vi "FPGA Main Default.vi"() -> (0 "ENC.B.CNTR 2":u32)   [LabVIEW 2017]
doc: "The myRIO v1.1 FPGA Shipping Personality. This personality contains support for:\n- 2 Analog Input Interrupt channel\n- 4 Digital Input Interrupt channel\n- 1 Timer\n- 1 Accelerometer\n- 1 Button\n- 4 LED\n- 10 Analog Input channels with 1 Sample\n- 6 Analog Output channels with 1 Sample\n- 40 Digital I/O channels with 1 Sample\n- 2 I2C channels\n- 4 Encoder channels\n- 6 PWM channels\n- 2 SPI channels"
uses:
  Sub VIs/Utilities/Start Boolean.ctl
  <vilib>/Platform/TimedLoop/XDataNode/timing_clust.ctl
  <vilib>/Platform/TimedLoop/XDataNode/nitl_modes.ctl
  <vilib>/Platform/TimedLoop/XDataNode/wakeup.ctl
  <vilib>/rvi/Emulation/niFpgaGetClockAttributes.vi
  <vilib>/rvi/Emulation/niFpgaSctlEmulationGetInTimedLoop.vi
  <vilib>/rvi/Emulation/niFpgaEmulationReportErrorSimple.vi
  <vilib>/rvi/eio/common/nirviEmuTemplateMethod_errors.vi
  <vilib>/rvi/Emulation/niFpgaCriticalErrorInLSC.vi
  <vilib>/rvi/Emulation/niFpgaProcessEmulError.vi
  <vilib>/rvi/Emulation/niFpgaEmulationIsFPGAContextNoSignature.vi
  <vilib>/rvi/errors/niFpgaSetErrorForExecOnDevCompSimple.vi
  <vilib>/rvi/eio/common/nirviEmuReportErrorAndStop.vi
  <vilib>/rvi/DataTransferAndStorage/Container/Common/niFpgaContainerGetUniqueNameForEmu.vi
  <vilib>/rvi/FIFO/Fifo_Resource/nirvififoEmulationSetSize.vi
  <vilib>/rvi/FIFO/Fifo_Resource/nirviFifoEmulationQueueMgr.vi
  <instcachedir>/0/nirviFifoEmulationQueueMgr_E5CAEC123FF24DC58D834DCA3CDAA9B5.lvgen/nirviFifoEmulationQueueMgr_E5CAEC123FF24DC58D834DCA3CDAA9B5_001.vi
  <vilib>/rvi/FIFO/Fifo_Resource/nirvififoEmulationDetermineInputValidOut.vi
  <vilib>/rvi/FIFO/Fifo_Resource/nirvififoEmulationCreateLock.vi
  <vilib>/rvi/FIFO/Fifo_Resource/nirvififoEmulationObtainLock.vi
  <vilib>/rvi/FIFO/Fifo_Resource/nirvififoEmulationReleaseLock.vi
  <vilib>/rvi/occurrence/nirviWaitOnOccurrenceBase.vi
  <vilib>/rvi/errors/nirviReportUnexpectedCaseInternalError.vi
  <vilib>/rvi/errors/nirviReportUnexpectedCaseInternalError (U32).vi
  <vilib>/Utility/error.llb/Clear Errors.vi
  <vilib>/rvi/DataTransferAndStorage/Container/Common/niFpgaContainerSetEmuInfo.vi
  <vilib>/eio/EIONode/EIONode.xnode
  <vilib>/rvi/DataTransferAndStorage/Container/XNode/niFpgaContainer.xnode
  <vilib>/rvi/FIFO/Fifo_Resource/nirvififoEmulationWrite.vi
  <vilib>/rvi/FIFO/Fifo_Resource/nirvififoEmulationRead.vi
  <vilib>/Platform/TimedLoop/XDataNode/XDataNode.xnode
  <vilib>/rvi/LocalResourceManager/LocalResourceManager.xnode
  <vilib>/Platform/TimedLoop/XDataNode/XDNodeRunTimeDep.lvlib
panel:
  out "ENCA.STAT.3 3":u8
  out "ENCA.STAT.3 2":u8
  out "ENCA.STAT.2":u8
  out "ENCA.STAT.3":u8
  out "ENCA.CNTR.3":u32
  out "ENC.A.CNTR.2":u32
  out "ENC.B.CNTR_4":u32
  in  "AO.A_0.VAL":u16
  in  "AO.A_1.VAL":u16
  in  "AO.B_0.VAL":u16
  in  "AO.B_1.VAL":u16
  out "AI.B_3.VAL":u16
  out "AI.B_2.VAL":u16
  out "AI.B_1.VAL":u16
  out "AI.B_0.VAL":u16
  out "AI.A_3.VAL":u16
  out "AI.A_2.VAL":u16
  out "AI.A_1.VAL":u16
  out "AI.A_0.VAL":u16
  out "DIO.B_7:0.IN":u8 format="%08b"
  in  "DIO.B_7:0.DIR":u8 format="%08b"
  in  "DIO.B_7:0.OUT":u8 format="%08b"
  in  "PWM.A_2.CS":u8=1
  in  "PWM.A_2.CNFG":u8=4
  out "PWM.A_2.CNTR":u16
  in  "PWM.A_2.MAX":u16=39999
  in  "PWM.A_2.CMP":u16=20000
  in  "PWM.A_1.CS":u8=1
  in  "PWM.A_1.CNFG":u8=4
  out "PWM.A_1.CNTR":u16
  in  "PWM.A_1.MAX":u16=39999
  in  "PWM.A_1.CMP":u16=20000
  in  "PWM.A_0.CS":u8=1
  in  "PWM.A_0.CNFG":u8=4
  out "PWM.A_0.CNTR":u16
  in  "PWM.A_0.CMP":u16=20000
  in  "PWM.A_0.MAX":u16=39999
  in  "SPI.A.DATO":u16
  out "SPI.A.DATI":u16
  in  "SPI.A.CNFG":u16=112
  in  "SPI.A.CNT":u16=19
  in  "SPI.B.CNT":u16=19
  in  "SPI.B.CNFG":u16=112 format="%0.0f"
  out "SPI.B.DATI":u16
  in  "SPI.B.DATO":u16
  out "ENC.A.CNTR":u32
  out "ENC.B.CNTR":u32
  out "ENC.A.STAT":u8 format="%08b"
  out "ENC.B.STAT":u8 format="%08b"
  in  "SPI.A.GO":T1
  out "SPI.A.STAT":u8 format="%08b"
  in  "SPI.B.GO":T1
  out "SPI.B.STAT":u8 format="%08b"
  out "I2C.B.STAT":u8 format="%08b"
  in  "I2C.B.CNTL":u8 format="%08b"
  out "I2C.A.STAT":u8 format="%08b"
  in  "I2C.A.CNTL":u8 format="%08b"
  in  "I2C.B.CNTR":u8=213
  in  "I2C.B.ADDR":u8 format="%08.0f"
  out "I2C.B.DATI":u8
  in  "I2C.B.DATO":u8
  in  "I2C.A.CNTR":u8=213
  in  "I2C.A.ADDR":u8 format="%08b"
  out "I2C.A.DATI":u8
  in  "I2C.A.DATO":u8
  in  "I2C.B.CNFG":u8=1 format="%08b"
  in  "I2C.A.CNFG":u8=1 format="%08b"
  in  "I2C.A.GO":T1
  in  "I2C.B.GO":T1
  out "SYS.AI.RDY":bool
  out "SYS.RDY":bool
  in  "PWM.B_2.CS":u8=1
  in  "PWM.B_2.CNFG":u8=4
  out "PWM.B_2.CNTR":u16
  in  "PWM.B_2.MAX":u16=39999
  in  "PWM.B_2.CMP":u16=20000
  in  "PWM.B_1.CS":u8=1
  in  "PWM.B_1.CNFG":u8=4
  out "PWM.B_1.CNTR":u16
  in  "PWM.B_1.MAX":u16=39999
  in  "PWM.B_1.CMP":u16=20000
  in  "PWM.B_0.CS":u8=1
  in  "PWM.B_0.CNFG":u8=4
  out "PWM.B_0.CNTR":u16
  in  "PWM.B_0.MAX":u16=39999
  in  "PWM.B_0.CMP":u16=20000
  out "DIO.A_7:0.IN":u8 format="%08b"
  in  "DIO.A_7:0.OUT":u8 format="%08b"
  in  "DIO.A_7:0.DIR":u8 format="%08b"
  out "DIO.C_7:0.IN":u8 format="%08b"
  in  "DIO.C_7:0.DIR":u8 format="%08b"
  in  "DIO.C_7:0.OUT":u8 format="%08b"
  out "AI.C_1.VAL":u16
  out "AI.C_0.VAL":u16
  in  "AO.C_0.VAL":u16
  in  "AO.C_1.VAL":u16
  in  "SYS.SELECTB":u8 format="%08b"
  in  "SYS.SELECTC":u8 format="%08b"
  in  "SYS.SELECTA":u8 format="%08b"
  out "ENC.C_0.CNTR":u32
  out "ENC.C_0.STAT":u8 format="%08b"
  out "ENC.C_1.CNTR":u32
  out "ENC.C_1.STAT":u8 format="%08b"
  in  "PWM.C_1.CS":u8=1
  in  "PWM.C_1.CNFG":u8=4
  out "PWM.C_1.CNTR":u16
  in  "PWM.C_1.CMP":u16=20000
  in  "PWM.C_1.MAX":u16=39999
  in  "PWM.C_0.CS":u8=1
  in  "PWM.C_0.CNFG":u8=4
  out "PWM.C_0.CNTR":u16
  in  "PWM.C_0.CMP":u16=20000
  in  "PWM.C_0.MAX":u16=39999
  out "DIO.A_15:8.IN":u8 format="%08b"
  in  "DIO.A_15:8.OUT":u8 format="%08b"
  in  "DIO.A_15:8.DIR":u8 format="%08b"
  out "DIO.B_15:8.IN":u8 format="%08b"
  in  "DIO.B_15:8.DIR":u8 format="%08b"
  in  "DIO.B_15:8.OUT":u8 format="%08b"
  in  "AO.SYS.GO":T1
  out "ACC.X.VAL":u16
  out "ACC.Y.VAL":u16
  out "SYS.ACC.RDY":bool
  out "ACC.Z.VAL":u16
  in  "DO.LED3:0":u8 format="%04b"
  out "DI.BTN":u8 format="%08b"
  out "AO.SYS.STAT":bool
  in  "IRQ.AI_A_3:0.CNFG":u8 format="%.0b"
  in  "IRQ.AI_A_0.THRESHOLD":u16
  in  "IRQ.AI_A_1.THRESHOLD":u16
  in  "IRQ.AI_A_0.NO":u8
  in  "IRQ.AI_A_1.NO":u8
  in  "IRQ.DIO_A_7:0.ENA":u8 format="%08b"
  in  "IRQ.DIO_A_7:0.RISE":u8 format="%08b"
  in  "IRQ.DIO_A_7:0.FALL":u8 format="%08b"
  in  "IRQ.DIO_A_0.NO":u8
  in  "IRQ.DIO_A_1.NO":u8
  in  "IRQ.DIO_A_2.NO":u8
  in  "IRQ.DIO_A_3.NO":u8
  in  "IRQ.DIO_A_3.CNT":u32
  in  "IRQ.DIO_A_2.CNT":u32
  in  "IRQ.DIO_A_1.CNT":u32
  in  "IRQ.DIO_A_0.CNT":u32
  in  "IRQ.AI_A_1.HYSTERESIS":u16=17
  in  "IRQ.TIMER.WRITE":u32
  in  "IRQ.TIMER.SETTIME":T1
  out "IRQ.TIMER.READ":u32
  in  "SPI.A.IRQ.NO":u8=15
  in  "SPI.B.IRQ.NO":u8=15
  in  "IRQ.AI_A_0.HYSTERESIS":u16=17
  in  "IRQ.DI_BTN.ENA":bool
  in  "IRQ.DI_BTN.RISE":bool
  in  "IRQ.DI_BTN.FALL":bool
  in  "IRQ.DI_BTN.CNT":u32
  in  "IRQ.DI_BTN.NO":u8
  # "System"
  # "Onboard Devices"
  # "Connector A"
  # "Connector B"
  # "Connector C"
  # "Audio Connector"
  # "Accelerometer"
  # "Analog Input"
  # "Analog Output"
  # "Digital I/O"
  # "PWM"
  # "SPI Master"
  # "Analog Input"
  # "Analog Output"
  # "Digital I/O"
  # "PWM"
  # "SPI Master"
  # "Analog Input"
  # "Analog Output"
  # "Digital I/O"
  # "Counters / PWM"
  # "Analog Input"
  # "Analog Output"
  # "IO Configuration"
  # "IO Configuration"
  # "IO Configuration"
  # "Encoders"
  # "Buttons & LEDs"
  # "Analog Interrupt"
  # "Digital Interrupt"
  # "Encoders"
  # "Encoders"
  # "Button Interrupt"
  # "I2C Master"
  # "I2C Master"
  # "Timer Interrupt"
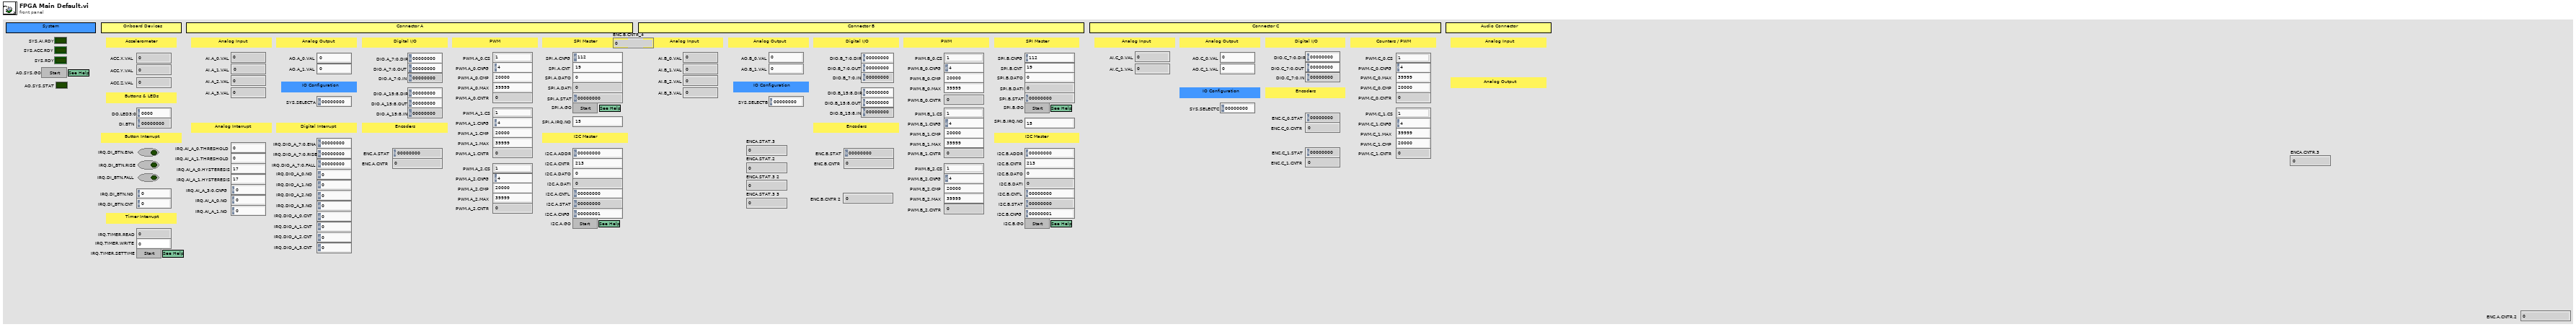
[diagram p1: front panel]
types:
  T1 = typedef "Start Boolean.ctl" = bool
  T2 = typedef "XDNodeRunTimeDep.lvlib/timing_clust.ctl" = cluster{"Expected End [f-1]":u64, "Actual End [f-1]":u64, "Finished Late? [f-1]":bool, "Expected End [i-1]":u64, "Actual End [i-1]":u64, "Finished Late? [i-1]":bool, "Expected Start [i]":u64, "Actual Start [i]":u64, "Expected Start [f]":u64, "Actual Start [f]":u64, "Source Name":string, "Structure Name":string, "Period":i64, "Deadline":i64, "Offset":i64, "Start":i64, "Priority":i32, "Timeout":i32, "Mode":T3, "Wakeup Reason":T4, "Error":errorcluster, "Source Type":string, "Secondary Source Type":string, "Global End Time":u64, "Global Start Time":u64, "Frame Duration":u64, "Iteration Duration":u64, "Assigned CPU":i32, "I/O Scan Engine Mode":u32}
  T3 = typedef "XDNodeRunTimeDep.lvlib/nitl_modes.ctl" = enum32{"No Change", "Process missed periods, maintain original phase", "Discard missed periods, maintain original phase", "Process missed periods, ignore original phase", "Discard missed periods, ignore original phase"}
  T4 = typedef "XDNodeRunTimeDep.lvlib/wakeup.ctl" = enum32{"Normal", "Aborted", "Asynchronous wakeup", "Timing source error", "Timed loop error", "Timeout"}
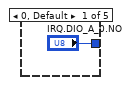
[diagram p9: hidden frame]
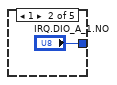
[diagram p10: hidden frame]
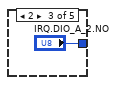
[diagram p11: hidden frame]
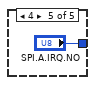
[diagram p12: hidden frame]
diagram:
  # "The Timed Loop does not allow writing the same FIFO outside the Timed Loop. Use another FIFO to push all interrupts from DIO in the Timed Loop to the IRQ Queue."
  # "The Timed Loop does not allow writing the same FIFO outside the Timed Loop. Use another FIFO to push all interrupts from Button in the Timed Loop to the IRQ Queue."
  # "The Timed Loop does not allow writing the same FIFO outside the Timed Loop. Use another FIFO to push all interrupts from DIO in the Timed Loop to the IRQ Queue."
  # "The accelerometer nodes take some time before the FPGA can first read the values. This is because it takes time to read from the accelerometer. An iteration of the While Loop will not complete until the accelerometer values have been read.\n\nAfter the completion of the first iteration of the While Loop, all indicators have valid values."
  # "The analog output nodes take some time before the FPGA write the values to the pins. The GO and STAT registers are used to handshake between the FPGA and host. When the host wants the values to be written, the host sets the GO register to TRUE. If the host reads the STAT register before setting the value of the GO register, it can wait for the value of the STAT register to invert. The value inversion tells the host that the output values have been written."
  # "The analog input nodes take some time before the FPGA can first read the values. This is because it takes time to set up the Analog-to-Digital converter (ADC) and convert the first reading. An iteration of the While Loop will not complete until all the analog input channels have been sampled.\n\nAfter the completion of the first iteration of the While Loop, all indicators have valid values."
  # "Note: On some hardware a \"ghosting effect\" may occur on any unconnected AI channels. For example, if channel AI0 is connected and channels AI1~AI7 are not connected the the value read at AI0 may be seen on indicators AI1~AI7. This is common for hardware that use a multiplexed (MUXed) Analog-to-Digital converter (ADC), because the input analog signal is used to charge a capacitor which does not discharge before the unconnected channel is read.\n\nYou can hide the \"ghosting effect\" by using an mask register. This register is used to decide when the indicator should be updated."
  # "The FPGA timer fires the interrupt request (IRQ) when TIMER.Read counts down to zero. If TIMER.Read is not zero, it counts down to one per microsecond."
  # "The only interface that sends interrupts to the RT side. Timer interrupts, analog input interrupts, digital input interrupts, and SPI interrupt share this interface.\n\nAll interrupts work in sequence. One interrupt waits until the previous interrupt request (IRQ) gets acknowledged on the RT side."
  # "NOTE: The SYS.RDY Boolean MUST exist and must become TRUE at some point. Otherwise, the myRIO VIs will not function correctly."
  # "There is some delay between the time when the FPGA code starts and the time when the analog inputs, accelerometer, and scaling values outputs are valid. If the host wants to ensure that there are valid values in theses registers it should wait for each subsystem to finish its initialization process. \n\nWhen all subsystems have finished initializinig, the SYS.RDY indicator turns true. The host can poll the SYS.RDY indicator to determine the status of the FPGA. Alternatively, the host can poll the individual SYS.xx.RDY indicators to determine the status of the individual subsystems.\n\nThis loop continues indefinitely, essentially making SYS.RDY a read-only register."
  n1 = while {
    stop <- FALSE stop-if-true
    # "Host Synchronization"
    n2 = local read "SYS.ACC.RDY"() -> (w13:bool)
    n3 = local read "SYS.AI.RDY"() -> (w15:bool)
    n4 = Compound Arithmetic op=AND(w15, w13) -> (→"SYS.RDY":bool)
  }
  n5 = while {
    stop <- FALSE stop-if-true
    # "Interrupt to RT"
    n6 = xnode ("FIFO Method Node")("Timeout"=-1) -> ("Element"=w18:u8)  [unwired: 1 in, 2 out]
    n7 = call <vilib>:"niFPGA Interrupt.vi"("Wait Until Cleared (F)"=TRUE, "IRQ Number (0)"=w18) -> ()  [unwired: 1 in]
  }
  n8 = while {
    stop <- FALSE stop-if-true
    # "Timer"
    n9 = local read "IRQ.TIMER.READ"() -> (w23:u32)
    n10 = Select(t="IRQ.TIMER.WRITE", s="IRQ.TIMER.SETTIME", f=w23) -> (s? t:f=w21:u32)
    n11 = case shown="Default" w21 {
      selector: w21 -> [w27 w30]
      tunnel: [w27 w28] -> w20
      frame 0 {
      }
      frame Default {
        n12 = Decrement(x=w30) -> (x-1=w29:u32)
        n13 = case shown="0" w29 {
          selector: w29 -> [w31 w34]
          tunnel: [w31 w34] -> w28
          frame Default {
          }
          frame 0 {
            w33 = u8 0  # Reserved for Timer IRQ
            n14 = xnode ("FIFO Method Node")("Element"=w33, "Timeout"=-1) -> ()  [unwired: 1 in, 2 out]
          }
        }
      }
    }
    "IRQ.TIMER.READ" <- w20
    n15 = call "Loop Timer"("Count(uSec)"=u8 1 ("Count(mSec)")) -> ()  [unwired: 1 out]
  }
  n16 = xnode "VI-Defined FIFO Configuration"() -> ("FIFO Out"=w3:refnum<k21>)
  n17 = while {
    tunnel: w3 -> [w36]
    i -> [w59]
    stop <- FALSE stop-if-true
    # "Analog Input"
    n18 = xnode "FPGA I/O Node"() -> ("ConnectorA/AI0"=w41:u16, "ConnectorA/AI1"=w40:u16, "ConnectorA/AI2"=→"AI.A_2.VAL":u16, "ConnectorA/AI3"=→"AI.A_3.VAL":u16, "ConnectorB/AI0"=→"AI.B_0.VAL":u16, "ConnectorB/AI1"=→"AI.B_1.VAL":u16, "ConnectorB/AI2"=→"AI.B_2.VAL":u16, "ConnectorB/AI3"=→"AI.B_3.VAL":u16, "ConnectorC/AI0"=w53:i16, "ConnectorC/AI1"=w52:i16)  [unwired: 10 in, 10 out]
    "AI.A_0.VAL" <- w41
    "AI.A_1.VAL" <- w40
    n19 = Greater Than 0?(x=w59) -> (x > 0?=→"SYS.AI.RDY":bool)
    n20 = Number To Boolean Array(number="IRQ.AI_A_3:0.CNFG") -> (Boolean array=w51:bool[])
    n21 = Index Array(array=w51) -> (element #1=w49:bool, element #2=w48:bool, element #3=w46:bool, element #4=w45:bool)  [unwired: 4 in]
    n22 = To Unsigned Word Integer(number=w53) -> (unsigned 16bit integer=→"AI.C_0.VAL":u16)
    n23 = To Unsigned Word Integer(number=w52) -> (unsigned 16bit integer=→"AI.C_1.VAL":u16)
    n24 = call "Check AI IRQ.vi"("Hysteresis"="IRQ.AI_A_1.HYSTERESIS", "FIFO In"=w36, "IRQ Number"="IRQ.AI_A_1.NO", "Threshold"="IRQ.AI_A_1.THRESHOLD", "Analog Value"=w40, "Rising Edge?"=w45, "Enable Interrupt?"=w46) -> ()  [unwired: 5 in]
    n25 = call "Check AI IRQ.vi"("Hysteresis"="IRQ.AI_A_0.HYSTERESIS", "FIFO In"=w36, "IRQ Number"="IRQ.AI_A_0.NO", "Threshold"="IRQ.AI_A_0.THRESHOLD", "Analog Value"=w41, "Rising Edge?"=w48, "Enable Interrupt?"=w49) -> ()  [unwired: 5 in]
  }
  n26 = while {
    stop <- FALSE stop-if-true
    # "Analog Output"
    n27 = feedback #1(FALSE) -> (w65:bool)
    n28 = case shown="True" "AO.SYS.GO" {
      tunnel: "AO.C_0.VAL" -> [_ w81]
      tunnel: "AO.C_1.VAL" -> [_ w80]
      tunnel: "AO.A_0.VAL" -> [_ w85]
      tunnel: "AO.A_1.VAL" -> [_ w84]
      tunnel: "AO.B_0.VAL" -> [_ w83]
      tunnel: "AO.B_1.VAL" -> [_ w82]
      tunnel: w65 -> [w74 w77]
      tunnel: [w74 w75] -> w63
      frame False {
      }
      frame True {
        n29 = To Word Integer(number=w81) -> (16bit integer=w79:i16)
        n30 = To Word Integer(number=w80) -> (16bit integer=w78:i16)
        n31 = flat-sequence {
          tunnel: w85 -> [w92]
          tunnel: w84 -> [w91]
          tunnel: w83 -> [w90]
          tunnel: w82 -> [w89]
          tunnel: w79 -> [w88]
          tunnel: w78 -> [w87]
          tunnel: w77 -> [w86]
          tunnel: [w86] -> w76
          tunnel: w76 -> [w94]
          tunnel: [w93] -> w75
          frame #0 {
            n32 = xnode "FPGA I/O Node"("ConnectorA/AO0"=w92, "ConnectorA/AO1"=w91, "ConnectorB/AO0"=w90, "ConnectorB/AO1"=w89, "ConnectorC/AO0"=w88, "ConnectorC/AO1"=w87) -> ()  [unwired: 6 in, 6 out]
          }
          frame #1 {
            n33 = Not(x=w94) -> (.not. x?=w93:bool)
          }
        }
      }
    }
    "AO.SYS.STAT" <- w63
    n34 = feedback-in #1(w63) -> ()
  }
  n35 = while {
    i -> [w99]
    stop <- FALSE stop-if-true
    # "Onboard Accelerometer"
    n36 = xnode "FPGA I/O Node"() -> ("AccelerationX"=w102:i16, "AccelerationY"=w101:i16, "AccelerationZ"=w100:i16)  [unwired: 3 in, 3 out]
    n37 = Greater Than 0?(x=w99) -> (x > 0?=→"SYS.ACC.RDY":bool)
    n38 = To Unsigned Word Integer(number=w102) -> (unsigned 16bit integer=→"ACC.X.VAL":u16)
    n39 = To Unsigned Word Integer(number=w101) -> (unsigned 16bit integer=→"ACC.Y.VAL":u16)
    n40 = To Unsigned Word Integer(number=w100) -> (unsigned 16bit integer=→"ACC.Z.VAL":u16)
  }
  n41 = xnode "VI-Defined FIFO Configuration"() -> ("FIFO Out"=w2:refnum<k21>)
  n42 = node-c288() -> (w5:T2)  [unwired: 1 in]
  n43 = timed-loop {
    timing: w5 -> [_]
    timing-out: [_] -> w4
    tunnel: w2 -> [w106]
    stop <- _ stop-if-true
    # "Onboard DIO"
    n44 = xnode "FPGA I/O Node"() -> ("Button0"=w110:bool)  [unwired: 1 in, 1 out]
    n45 = Number To Boolean Array(number="DO.LED3:0") -> (Boolean array=w115:bool[])
    n46 = Build Array(w110) -> (w118:bool[])
    n47 = Index Array(array=w115) -> (element #1=w114:bool, element #2=w113:bool, element #3=w112:bool, element #4=w111:bool)  [unwired: 4 in]
    n48 = call "DIO IRQ 1-bit.vi"("IRQ.NO"="IRQ.DI_BTN.NO", "IRQ.CNT"="IRQ.DI_BTN.CNT", "FIFO in"=w106, "IRQ.FALL"="IRQ.DI_BTN.FALL", "IRQ.RISE"="IRQ.DI_BTN.RISE", "IRQ.ENA"="IRQ.DI_BTN.ENA", "DIO"=w110) -> ()  [unwired: 5 in]
    n49 = Boolean Array To Number(Boolean array=w118) -> (number=→"DI.BTN":u8)
    n50 = xnode "FPGA I/O Node"("LED0"=w114, "LED1"=w113, "LED2"=w112, "LED3"=w111) -> ()  [unwired: 4 in, 4 out]
  }
  n51 = while {
    stop <- FALSE stop-if-true
    # "Button SCTL Interrupt Buffer"
    n52 = feedback #2(u8 0 ("Element")) -> (w123:u8)
    n53 = feedback #3(FALSE ("Timed Out?")) -> (w127:bool)
    n54 = case shown="False" w127 {
      tunnel: [w129 w131] -> w124
      tunnel: w123 -> [_ w131]
      frame False {
        n55 = xnode ("FIFO Method Node")("Timeout"=-1) -> ("Element"=w129:u8)  [unwired: 1 in, 2 out]
      }
      frame True {
      }
    }
    n56 = feedback-in #2(w124) -> ()
    n57 = xnode ("FIFO Method Node")("Element"=w124, "Timeout"=0) -> ("Timed Out?"=w125:bool)  [unwired: 1 in, 1 out]
    n58 = feedback-in #3(w125) -> ()
  }
  n59 = node-c288(w4) -> ()
  n60 = node-c288() -> (w9:T2)  [unwired: 1 in]
  n61 = xnode "VI-Defined FIFO Configuration"() -> ()  [unwired: 1 out]
  n62 = while {
    stop <- FALSE stop-if-true
    # "Connector A SCTL Interrupt Buffer"
    n63 = feedback #4(u8 0 ("Element")) -> (w134:u8)
    n64 = feedback #5(FALSE ("Timed Out?")) -> (w138:bool)
    n65 = case shown="False" w138 {
      tunnel: [w140 w142] -> w135
      tunnel: w134 -> [_ w142]
      frame False {
        n66 = xnode ("FIFO Method Node")("Timeout"=-1) -> ("Element"=w140:u8)  [unwired: 1 in, 2 out]
      }
      frame True {
      }
    }
    n67 = feedback-in #4(w135) -> ()
    n68 = xnode ("FIFO Method Node")("Element"=w135, "Timeout"=0) -> ("Timed Out?"=w136:bool)  [unwired: 1 in, 1 out]
    n69 = feedback-in #5(w136) -> ()
  }
  n70 = timed-loop {
    timing: w9 -> [_]
    timing-out: [_] -> w8
    stop <- _ stop-if-true
    w201 = u16 5 ("Debounce Ticks")
    w202 = u8 0
    # "Importante notar que \nNO es posible usar DIO2 \nDIO3 como encoders"
    # "Este es el cambio que hice. En lugar de usar los conectores \nB/DIO2 como entradas salida, use el B/DIO0 y 1 como encoders"
    # "Trigger the interrupt at next \ntick if timeout"
    # "DIO / Encoder"
    # "DIO / I2C Master"
    # "DIO / PWM"
    # "ENCODERS"
    # "DIO/ SPI Master"
    # "Connector A DIO"
    n71 = call "Split HDC Bank1 DIO.vi"("IN 7:0"="DIO.A_7:0.OUT") -> ("OUT 3:0"=w160:fxp<+,4,4>, "OUT 4"=w158:bool, "OUT 7:5"=w320:fxp<+,3,3>)
    n72 = Number To Boolean Array(number=w160) -> (Boolean array=w191:bool[])
    n73 = Index Array(array=w191) -> (element #1=w190:bool, element #2=w189:bool, element #3=w188:bool, element #4=w187:bool)  [unwired: 4 in]
    n74 = Build Array(w188, w187) -> (w185:bool[])
    n75 = Build Array(w190, w189) -> (w186:bool[])
    n76 = call "Split HDC Bank1 DIO.vi"("IN 7:0"="DIO.A_7:0.DIR") -> ("OUT 3:0"=w159:fxp<+,4,4>, "OUT 4"=w157:bool, "OUT 7:5"=w319:fxp<+,3,3>)
    n77 = Number To Boolean Array(number=w159) -> (Boolean array=w183:bool[])
    n78 = Index Array(array=w183) -> (element #1=w182:bool, element #2=w181:bool, element #3=w180:bool, element #4=w179:bool)  [unwired: 4 in]
    n79 = Build Array(w180, w179) -> (w177:bool[])
    n80 = Build Array(w182, w181) -> (w178:bool[])
    n81 = call "Split HDC Function Select.vi"("IN 7:0"="SYS.SELECTA") -> ("OUT 1:0"=w269:fxp<+,2,2>, "OUT 7"=w265:bool, "OUT 2"=w268:bool, "OUT 3"=w267:bool, "OUT 4"=w266:bool)  [unwired: 1 out]
    n82 = Boolean Array To Number(Boolean array=w178) -> (number=w176:fxp<+,2,2>)
    n83 = Boolean Array To Number(Boolean array=w186) -> (number=w184:fxp<+,2,2>)
    n84 = Boolean Array To Number(Boolean array=w185) -> (number=w147:fxp<+,2,2>)
    n85 = Boolean Array To Number(Boolean array=w177) -> (number=w148:fxp<+,2,2>)
    n86 = call "DIO 2-bit.vi"("DIO0 Refnum"=refnum<k21> "ConnectorA/DIO2" ("DIO2 Refnum"), "DIR 1:0"=w148, "OUT 1:0"=w147, "DIO1 Refnum"=refnum<k21> "ConnectorA/DIO3" ("DIO3 Refnum")) -> ("IN 1:0"=w151:fxp<+,2,2>)  [unwired: 7 in]
    n87 = call "DIO_Encoder.vi"("DIO.1:0.OUT"=w184, "DIO.1:0.DIR"=w176, "QE.CNFG"=u8 1, "DIO.1/QE.B"=refnum<k21> "ConnectorA/DIO1" ("DIO1 Refnum"), "SELECT"=TRUE, "DIO.0/QE.A"=refnum<k21> "ConnectorA/DIO0" ("DIO0 Refnum")) -> ("DIO.1:0.IN"=w199:fxp<+,2,2>, "QE.CNTR"=→"ENC.A.CNTR.2":u32, "QE.STAT"=→"ENCA.STAT.2":u8)  [unwired: 11 in]
    n88 = call "DIO_SPI.vi"("DIO.2:0.OUT"=w320, "DIO.2:0.DIR"=w319, "SPI.CNT"="SPI.A.CNT", "SPI.CNFG"="SPI.A.CNFG", "SPI.DATO"="SPI.A.DATO", "SPI.GO"="SPI.A.GO", "DIO.2/SPI.MOSI Refnum"=refnum<k21> "ConnectorA/DIO7" ("DIO.2/SPI.SCLK"), "SELECT.1:0"=w269, "DIO.1/SPI.MISO Refnum"=refnum<k21> "ConnectorA/DIO6" ("DIO.1/SPI.MOSI"), "DIO.0/SPI.SCLK Refnum"=refnum<k21> "ConnectorA/DIO5" ("DIO.0/SPI.MISO")) -> ("DIO.2:0.IN"=w301:fxp<+,3,3>, "SPI.DATI"=→"SPI.A.DATI":u16, "SPI.STAT"=w209:u8)  [unwired: 7 in]
    "SPI.A.STAT" <- w209
    n89 = Number To Boolean Array(number=w209) -> (Boolean array=w211:bool[])
    n90 = Index Array(array=w211) -> (element=w210:bool)  [unwired: 1 in]
    n91 = Number To Boolean Array(number=w199) -> (Boolean array=w198:bool[])
    n92 = call "Falling Edge Trigger.vi"("Signal"=w210) -> ("Trigger?"=w208:bool)
    n93 = Number To Boolean Array(number=w151) -> (Boolean array=w173:bool[])
    n94 = Index Array(array=w198) -> (element #1=w197:bool, element #2=w196:bool)  [unwired: 2 in]
    n95 = Index Array(array=w173) -> (element #1=w175:bool, element #2=w174:bool)  [unwired: 2 in]
    n96 = Build Array(w197, w196, w175, w174) -> (w195:bool[])
    n97 = Boolean Array To Number(Boolean array=w195) -> (number=w152:fxp<+,4,4>)
    n98 = Number To Boolean Array(number=w152) -> (Boolean array=w246:bool[])
    n99 = Number To Boolean Array(number="IRQ.DIO_A_7:0.ENA") -> (Boolean array=w252:bool[])
    n100 = Number To Boolean Array(number="IRQ.DIO_A_7:0.RISE") -> (Boolean array=w251:bool[])
    n101 = Number To Boolean Array(number="IRQ.DIO_A_7:0.FALL") -> (Boolean array=w250:bool[])
    n102 = call "Split HDC Bank2 DIO.vi"("IN 7:0"="DIO.A_15:8.OUT") -> ("OUT 5"=w156:bool, "OUT 7:6"=w273:fxp<+,2,2>, "OUT 4:3"=w254:fxp<+,2,2>, "OUT 2"=w256:bool, "OUT 0"=w260:bool, "OUT 1"=w259:bool)  [unwired: 2 in]
    n103 = Build Array(w158, w156) -> (w169:bool[])
    n104 = Boolean Array To Number(Boolean array=w169) -> (number=w168:fxp<+,2,2>)
    n105 = call "Split HDC Bank2 DIO.vi"("IN 7:0"="DIO.A_15:8.DIR") -> ("OUT 5"=w155:bool, "OUT 7:6"=w272:fxp<+,2,2>, "OUT 4:3"=w253:fxp<+,2,2>, "OUT 2"=w255:bool, "OUT 0"=w258:bool, "OUT 1"=w257:bool)  [unwired: 2 in]
    n106 = Build Array(w157, w155) -> (w166:bool[])
    n107 = Boolean Array To Number(Boolean array=w166) -> (number=w167:fxp<+,2,2>)
    n108 = call "DIO_Encoder.vi"("DIO.1:0.OUT"=w168, "DIO.1:0.DIR"=w167, "QE.CNFG"=u8 1, "DIO.1/QE.B"=refnum<k21> "ConnectorA/DIO13" ("DIO Refnum"), "SELECT"=TRUE, "DIO.0/QE.A"=refnum<k21> "ConnectorA/DIO4" ("DIO Refnum")) -> ("DIO.1:0.IN"=w161:fxp<+,2,2>, "QE.CNTR"=→"ENCA.CNTR.3":u32, "QE.STAT"=→"ENCA.STAT.3":u8)  [unwired: 11 in]
    n109 = Number To Boolean Array(number=w161) -> (Boolean array=w162:bool[])
    n110 = Index Array(array=w162) -> (element #1=w154:bool, element #2=w153:bool)  [unwired: 2 in]
    n111 = call "Join HDC Bank1 DIO.vi"("IN 7:5"=w301, "IN 4"=w154, "IN 3:0"=w152) -> ("OUT 7:0"=→"DIO.A_7:0.IN":u8)
    n112 = Index Array(array=w246) -> (element #1=w227:bool, element #2=w242:bool, element #3=w241:bool, element #4=w240:bool)  [unwired: 4 in]
    n113 = Index Array(array=w252) -> (element #1=w245:bool, element #2=w239:bool, element #3=w238:bool, element #4=w237:bool)  [unwired: 4 in]
    n114 = Index Array(array=w251) -> (element #1=w244:bool, element #2=w236:bool, element #3=w235:bool, element #4=w234:bool)  [unwired: 4 in]
    n115 = Index Array(array=w250) -> (element #1=w243:bool, element #2=w233:bool, element #3=w232:bool, element #4=w231:bool)  [unwired: 4 in]
    n116 = call "Check DI IRQ.vi"("Debounce Ticks"=w201, "Count"="IRQ.DIO_A_0.CNT", "On Falling Edge?"=w243, "On Rising Edge?"=w244, "Enable Interrupt?"=w245, "Digital In"=w227) -> ("Trigger?"=w221:bool)  [unwired: 5 in]
    n117 = call "Check DI IRQ.vi"("Debounce Ticks"=w201, "Count"="IRQ.DIO_A_1.CNT", "On Falling Edge?"=w233, "On Rising Edge?"=w236, "Enable Interrupt?"=w239, "Digital In"=w242) -> ("Trigger?"=w220:bool)  [unwired: 5 in]
    n118 = call "Check DI IRQ.vi"("Debounce Ticks"=w201, "Count"="IRQ.DIO_A_2.CNT", "On Falling Edge?"=w232, "On Rising Edge?"=w235, "Enable Interrupt?"=w238, "Digital In"=w241) -> ("Trigger?"=w219:bool)  [unwired: 5 in]
    n119 = call "DIO_PWM.vi"("DIO.OUT"=w260, "DIO.DIR"=w258, "PWM.CS"="PWM.A_0.CS", "PWM.CNFG"="PWM.A_0.CNFG", "PWM.CMP"="PWM.A_0.CMP", "PWM.MAX"="PWM.A_0.MAX", "DIO/PWM"=refnum<k21> "ConnectorA/DIO8", "SELECT"=w268) -> ("DIO.IN"=w264:bool, "PWM.CNTR"=→"PWM.A_0.CNTR":u16)  [unwired: 10 in]
    n120 = call "DIO_PWM.vi"("DIO.OUT"=w259, "DIO.DIR"=w257, "PWM.CS"="PWM.A_1.CS", "PWM.CNFG"="PWM.A_1.CNFG", "PWM.CMP"="PWM.A_1.CMP", "PWM.MAX"="PWM.A_1.MAX", "DIO/PWM"=refnum<k21> "ConnectorA/DIO9", "SELECT"=w267) -> ("DIO.IN"=w263:bool, "PWM.CNTR"=→"PWM.A_1.CNTR":u16)  [unwired: 10 in]
    n121 = call "DIO_PWM.vi"("DIO.OUT"=w256, "DIO.DIR"=w255, "PWM.CS"="PWM.A_2.CS", "PWM.CNFG"="PWM.A_2.CNFG", "PWM.CMP"="PWM.A_2.CMP", "PWM.MAX"="PWM.A_2.MAX", "DIO/PWM"=refnum<k21> "ConnectorA/DIO10", "SELECT"=w266) -> ("DIO.IN"=w262:bool, "PWM.CNTR"=→"PWM.A_2.CNTR":u16)  [unwired: 10 in]
    n122 = call "Check DI IRQ.vi"("Debounce Ticks"=w201, "Count"="IRQ.DIO_A_3.CNT", "On Falling Edge?"=w231, "On Rising Edge?"=w234, "Enable Interrupt?"=w237, "Digital In"=w240) -> ("Trigger?"=w218:bool)  [unwired: 5 in]
    n123 = feedback #6(w202) -> (w204:u8)
    n124 = Less?(x=w204, y=4 ("x")) -> (x < y?=w206:bool)
    n125 = Increment(x=w204) -> (x+1=w205:u8)
    n126 = Select(t=w205, s=w206, f=w202) -> (s? t:f=w203:u8)
    n127 = feedback-in #6(w203) -> ()
    n128 = case shown="3" w204 {
      tunnel: ["IRQ.DIO_A_0.NO" "IRQ.DIO_A_1.NO" "IRQ.DIO_A_2.NO" "IRQ.DIO_A_3.NO" "SPI.A.IRQ.NO"] -> w230
      frame 0, Default {
      }
      frame 1 {
      }
      frame 2 {
      }
      frame 3 {
      }
      frame 4 {
      }
    }
    n129 = Build Array(w221, w220, w219, w218, w208) -> (w216:bool[])
    n130 = call "DIO_Encoder.vi"("DIO.1:0.OUT"=w254, "DIO.1:0.DIR"=w253, "QE.CNFG"=u8 1, "DIO.1/QE.B"=refnum<k21> "ConnectorA/DIO12", "SELECT"=TRUE, "DIO.0/QE.A"=refnum<k21> "ConnectorA/DIO11") -> ("DIO.1:0.IN"=w261:fxp<+,2,2>, "QE.CNTR"=→"ENC.A.CNTR":u32, "QE.STAT"=→"ENC.A.STAT":u8)  [unwired: 11 in]
    n131 = call "DIO_I2C.vi"("DIO.1:0.OUT"=w273, "DIO.1:0.DIR"=w272, "I2C.CNFG"="I2C.A.CNFG", "I2C.CNTL"="I2C.A.CNTL", "I2C.ADDR"="I2C.A.ADDR", "I2C.DATO"="I2C.A.DATO", "DIO.1/I2C.SDA"=refnum<k21> "ConnectorA/DIO15" ("DIO.1/I2C.SCL"), "I2C.CNTR"="I2C.A.CNTR", "DIO.0/I2C.SCL"=refnum<k21> "ConnectorA/DIO14" ("DIO.0/I2C.SDA"), "Execute?"="I2C.A.GO", "SELECT"=w265) -> ("DIO.1:0.IN"=w271:fxp<+,2,2>, "I2C.DATI"=→"I2C.A.DATI":u8, "I2C.STAT"=→"I2C.A.STAT":u8)  [unwired: 6 in]
    n132 = feedback #7(bool[] [FALSE, FALSE, FALSE, FALSE, FALSE] ("initialized array")) -> (w212:bool[])
    n133 = Or(x=w216, y=w212) -> (x .or. y?=w217:bool[])
    n134 = Index Array(array=w217, index=w204) -> (element=w215:bool)
    n135 = case shown="True" w215 {
      selector: w215 -> [w321 _]
      tunnel: [w321 w322] -> w214
      tunnel: w230 -> [_ w323]
      frame False {
      }
      frame True {
        n136 = xnode ("FIFO Method Node")("Element"=w323, "Timeout"=0) -> ("Timed Out?"=w322:bool)  [unwired: 1 in, 1 out]
      }
    }
    n137 = Replace Array Subset(array=w217, new element=w214, index=w204) -> (w213:bool[])
    n138 = feedback-in #7(w213) -> ()
    n139 = call "Join HDC Bank2 DIO.vi"("IN 7:6"=w271, "IN 5"=w153, "IN 4:3"=w261, "IN 0"=w264, "IN 2"=w262, "IN 1"=w263) -> ("OUT 7:0"=→"DIO.A_15:8.IN":u8)  [unwired: 4 in]
  }
  n140 = node-c288(w8) -> ()
  n141 = xnode "VI-Defined FIFO Configuration"() -> ("FIFO Out"=w1:refnum<k21>)
  n142 = node-c288() -> (w7:T2)  [unwired: 1 in]
  n143 = timed-loop {
    timing: w7 -> [_]
    timing-out: [_] -> w6
    tunnel: w1 -> [w391]
    stop <- _ stop-if-true
    w342 = TRUE ("SELECT")
    w341 = u8 1 ("QE.CNFG")
    # "Importante notar que \nNO es posible usar DIO2 \nDIO3 como encoders"
    # "Este es el cambio que hice. En lugar de usar los conectores \nB/DIO2 como entradas salida, use el B/DIO0 y 1 como encoders"
    # "DIO / Encoder"
    # "DIO / I2C Master"
    # "DIO / PWM"
    # "ENCODERS"
    # "DIO/ SPI Master"
    # "Connector B DIO"
    n144 = call "Split HDC Bank1 DIO.vi"("IN 7:0"="DIO.B_7:0.OUT") -> ("OUT 3:0"=w378:fxp<+,4,4>, "OUT 4"=w354:bool, "OUT 7:5"=w380:fxp<+,3,3>)
    n145 = Number To Boolean Array(number=w378) -> (Boolean array=w379:bool[])
    n146 = Index Array(array=w379) -> (element #1=w377:bool, element #2=w376:bool, element #3=w375:bool, element #4=w374:bool)  [unwired: 4 in]
    n147 = Build Array(w375, w374) -> (w372:bool[])
    n148 = Build Array(w377, w376) -> (w373:bool[])
    n149 = call "Split HDC Bank1 DIO.vi"("IN 7:0"="DIO.B_7:0.DIR") -> ("OUT 3:0"=w362:fxp<+,4,4>, "OUT 4"=w350:bool, "OUT 7:5"=w370:fxp<+,3,3>)
    n150 = Number To Boolean Array(number=w362) -> (Boolean array=w369:bool[])
    n151 = Index Array(array=w369) -> (element #1=w368:bool, element #2=w367:bool, element #3=w366:bool, element #4=w365:bool)  [unwired: 4 in]
    n152 = Build Array(w366, w365) -> (w363:bool[])
    n153 = Build Array(w368, w367) -> (w364:bool[])
    n154 = call "Split HDC Function Select.vi"("IN 7:0"="SYS.SELECTB") -> ("OUT 1:0"=w446:fxp<+,2,2>, "OUT 7"=w442:bool, "OUT 2"=w445:bool, "OUT 3"=w444:bool, "OUT 4"=w443:bool)  [unwired: 1 out]
    n155 = Boolean Array To Number(Boolean array=w364) -> (number=w361:fxp<+,2,2>)
    n156 = Boolean Array To Number(Boolean array=w373) -> (number=w371:fxp<+,2,2>)
    n157 = Boolean Array To Number(Boolean array=w372) -> (number=w336:fxp<+,2,2>)
    n158 = Boolean Array To Number(Boolean array=w363) -> (number=w337:fxp<+,2,2>)
    n159 = call "DIO 2-bit.vi"("DIO0 Refnum"=refnum<k21> "ConnectorB/DIO2" ("DIO2 Refnum"), "DIR 1:0"=w337, "OUT 1:0"=w336, "DIO1 Refnum"=refnum<k21> "ConnectorB/DIO3" ("DIO3 Refnum")) -> ("IN 1:0"=w340:fxp<+,2,2>)  [unwired: 7 in]
    n160 = call "DIO_Encoder.vi"("DIO.1:0.OUT"=w371, "DIO.1:0.DIR"=w361, "QE.CNFG"=w341, "DIO.1/QE.B"=refnum<k21> "ConnectorB/DIO1" ("DIO1 Refnum"), "SELECT"=w342, "DIO.0/QE.A"=refnum<k21> "ConnectorB/DIO0" ("DIO0 Refnum")) -> ("DIO.1:0.IN"=w389:fxp<+,2,2>, "QE.CNTR"=→"ENC.B.CNTR 2":u32, "QE.STAT"=→"ENCA.STAT.3 2":u8)  [unwired: 11 in]
    n161 = call "DIO_SPI.vi"("DIO.2:0.OUT"=w380, "DIO.2:0.DIR"=w370, "SPI.CNT"="SPI.B.CNT", "SPI.CNFG"="SPI.B.CNFG", "SPI.DATO"="SPI.B.DATO", "SPI.GO"="SPI.B.GO", "DIO.2/SPI.MOSI Refnum"=refnum<k21> "ConnectorB/DIO7" ("DIO.2/SPI.SCLK"), "SELECT.1:0"=w446, "DIO.1/SPI.MISO Refnum"=refnum<k21> "ConnectorB/DIO6" ("DIO.1/SPI.MOSI"), "DIO.0/SPI.SCLK Refnum"=refnum<k21> "ConnectorB/DIO5" ("DIO.0/SPI.MISO")) -> ("DIO.2:0.IN"=w450:fxp<+,3,3>, "SPI.DATI"=→"SPI.B.DATI":u16, "SPI.STAT"=w392:u8)  [unwired: 7 in]
    "SPI.B.STAT" <- w392
    n162 = call "SPI IRQ.vi"("SPI.A.IRQ.NO"="SPI.B.IRQ.NO", "SPI.STAT"=w392, "FIFO In"=w391) -> ()  [unwired: 9 in]
    n163 = Number To Boolean Array(number=w389) -> (Boolean array=w388:bool[])
    n164 = Number To Boolean Array(number=w340) -> (Boolean array=w358:bool[])
    n165 = Index Array(array=w388) -> (element #1=w387:bool, element #2=w386:bool)  [unwired: 2 in]
    n166 = Index Array(array=w358) -> (element #1=w360:bool, element #2=w359:bool)  [unwired: 2 in]
    n167 = Build Array(w387, w386, w360, w359) -> (w385:bool[])
    n168 = Boolean Array To Number(Boolean array=w385) -> (number=w384:fxp<+,4,4>)
    n169 = call "Split HDC Bank2 DIO.vi"("IN 7:0"="DIO.B_15:8.OUT") -> ("OUT 5"=w352:bool, "OUT 7:6"=w449:fxp<+,2,2>, "OUT 4:3"=w402:fxp<+,2,2>, "OUT 2"=w403:bool, "OUT 0"=w405:bool, "OUT 1"=w404:bool)  [unwired: 2 in]
    n170 = Build Array(w354, w352) -> (w355:bool[])
    n171 = Boolean Array To Number(Boolean array=w355) -> (number=w353:fxp<+,2,2>)
    n172 = call "Split HDC Bank2 DIO.vi"("IN 7:0"="DIO.B_15:8.DIR") -> ("OUT 5"=w349:bool, "OUT 7:6"=w448:fxp<+,2,2>, "OUT 4:3"=w398:fxp<+,2,2>, "OUT 2"=w399:bool, "OUT 0"=w401:bool, "OUT 1"=w400:bool)  [unwired: 2 in]
    n173 = Build Array(w350, w349) -> (w348:bool[])
    n174 = Boolean Array To Number(Boolean array=w348) -> (number=w351:fxp<+,2,2>)
    n175 = call "DIO_Encoder.vi"("DIO.1:0.OUT"=w353, "DIO.1:0.DIR"=w351, "QE.CNFG"=w341, "DIO.1/QE.B"=refnum<k21> "ConnectorB/DIO13" ("DIO Refnum"), "SELECT"=w342, "DIO.0/QE.A"=refnum<k21> "ConnectorB/DIO4" ("DIO Refnum")) -> ("DIO.1:0.IN"=w345:fxp<+,2,2>, "QE.CNTR"=→"ENC.B.CNTR_4":u32, "QE.STAT"=→"ENCA.STAT.3 3":u8)  [unwired: 11 in]
    n176 = Number To Boolean Array(number=w345) -> (Boolean array=w346:bool[])
    n177 = Index Array(array=w346) -> (element #1=w344:bool, element #2=w343:bool)  [unwired: 2 in]
    n178 = call "Join HDC Bank1 DIO.vi"("IN 7:5"=w450, "IN 4"=w344, "IN 3:0"=w384) -> ("OUT 7:0"=→"DIO.B_7:0.IN":u8)
    n179 = call "DIO_PWM.vi"("DIO.OUT"=w405, "DIO.DIR"=w401, "PWM.CS"="PWM.B_0.CS", "PWM.CNFG"="PWM.B_0.CNFG", "PWM.CMP"="PWM.B_0.CMP", "PWM.MAX"="PWM.B_0.MAX", "DIO/PWM"=refnum<k21> "ConnectorB/DIO8", "SELECT"=w445) -> ("DIO.IN"=w397:bool, "PWM.CNTR"=→"PWM.B_0.CNTR":u16)  [unwired: 10 in]
    n180 = call "DIO_PWM.vi"("DIO.OUT"=w404, "DIO.DIR"=w400, "PWM.CS"="PWM.B_1.CS", "PWM.CNFG"="PWM.B_1.CNFG", "PWM.CMP"="PWM.B_1.CMP", "PWM.MAX"="PWM.B_1.MAX", "DIO/PWM"=refnum<k21> "ConnectorB/DIO9", "SELECT"=w444) -> ("DIO.IN"=w396:bool, "PWM.CNTR"=→"PWM.B_1.CNTR":u16)  [unwired: 10 in]
    n181 = call "DIO_PWM.vi"("DIO.OUT"=w403, "DIO.DIR"=w399, "PWM.CS"="PWM.B_2.CS", "PWM.CNFG"="PWM.B_2.CNFG", "PWM.CMP"="PWM.B_2.CMP", "PWM.MAX"="PWM.B_2.MAX", "DIO/PWM"=refnum<k21> "ConnectorB/DIO10", "SELECT"=w443) -> ("DIO.IN"=w395:bool, "PWM.CNTR"=→"PWM.B_2.CNTR":u16)  [unwired: 10 in]
    n182 = call "DIO_Encoder.vi"("DIO.1:0.OUT"=w402, "DIO.1:0.DIR"=w398, "QE.CNFG"=u8 1, "DIO.1/QE.B"=refnum<k21> "ConnectorB/DIO12", "SELECT"=TRUE, "DIO.0/QE.A"=refnum<k21> "ConnectorB/DIO11") -> ("DIO.1:0.IN"=w394:fxp<+,2,2>, "QE.CNTR"=→"ENC.B.CNTR":u32, "QE.STAT"=→"ENC.B.STAT":u8)  [unwired: 11 in]
    n183 = call "DIO_I2C.vi"("DIO.1:0.OUT"=w449, "DIO.1:0.DIR"=w448, "I2C.CNFG"="I2C.B.CNFG", "I2C.CNTL"="I2C.B.CNTL", "I2C.ADDR"="I2C.B.ADDR", "I2C.DATO"="I2C.B.DATO", "DIO.1/I2C.SDA"=refnum<k21> "ConnectorB/DIO15" ("DIO.1/I2C.SCL"), "I2C.CNTR"="I2C.B.CNTR", "DIO.0/I2C.SCL"=refnum<k21> "ConnectorB/DIO14" ("DIO.0/I2C.SDA"), "Execute?"="I2C.B.GO", "SELECT"=w442) -> ("DIO.1:0.IN"=w447:fxp<+,2,2>, "I2C.DATI"=→"I2C.B.DATI":u8, "I2C.STAT"=→"I2C.B.STAT":u8)  [unwired: 6 in]
    n184 = call "Join HDC Bank2 DIO.vi"("IN 7:6"=w447, "IN 5"=w343, "IN 4:3"=w394, "IN 0"=w397, "IN 2"=w395, "IN 1"=w396) -> ("OUT 7:0"=→"DIO.B_15:8.IN":u8)  [unwired: 4 in]
  }
  n185 = while {
    stop <- FALSE stop-if-true
    # "Connector B SCTL Interrupt Buffer"
    n186 = feedback #8(u8 0 ("Element")) -> (w465:u8)
    n187 = feedback #9(FALSE ("Timed Out?")) -> (w469:bool)
    n188 = case shown="False" w469 {
      tunnel: [w471 w473] -> w466
      tunnel: w465 -> [_ w473]
      frame False {
        n189 = xnode ("FIFO Method Node")("Timeout"=-1) -> ("Element"=w471:u8)  [unwired: 1 in, 2 out]
      }
      frame True {
      }
    }
    n190 = feedback-in #8(w466) -> ()
    n191 = xnode ("FIFO Method Node")("Element"=w466, "Timeout"=0) -> ("Timed Out?"=w467:bool)  [unwired: 1 in, 1 out]
    n192 = feedback-in #9(w467) -> ()
  }
  n193 = node-c288(w6) -> ()
  n194 = node-c288() -> (w11:T2)  [unwired: 1 in]
  n195 = timed-loop {
    timing: w11 -> [_]
    timing-out: [_] -> w10
    stop <- _ stop-if-true
    # "Connector C  DIO"
    n196 = call "Split myDAQ DIO.vi"("IN 7:0"="DIO.C_7:0.OUT") -> ("OUT 2, OUT0"=w496:fxp<+,2,2>, "OUT 1"=w495:bool, "OUT 3"=w494:bool, "OUT 7"=w491:bool, "OUT 6, OUT 4"=w493:fxp<+,2,2>, "OUT 5"=w492:bool)  [unwired: 4 in]
    n197 = call "Split myDAQ DIO.vi"("IN 7:0"="DIO.C_7:0.DIR") -> ("OUT 2, OUT0"=w490:fxp<+,2,2>, "OUT 1"=w489:bool, "OUT 3"=w488:bool, "OUT 7"=w485:bool, "OUT 6, OUT 4"=w487:fxp<+,2,2>, "OUT 5"=w486:bool)  [unwired: 4 in]
    n198 = call "Split myDAQ Function Select.vi"("IN 7:0"="SYS.SELECTC") -> ("OUT 1"=w500:bool, "OUT 3"=w499:bool)  [unwired: 2 in, 2 out]
    n199 = call "DIO_Encoder.vi"("DIO.1:0.OUT"=w496, "DIO.1:0.DIR"=w490, "QE.CNFG"=u8 1, "DIO.1/QE.B"=refnum<k21> "ConnectorC/DIO2", "SELECT"=TRUE, "DIO.0/QE.A"=refnum<k21> "ConnectorC/DIO0") -> ("DIO.1:0.IN"=w483:fxp<+,2,2>, "QE.CNTR"=→"ENC.C_0.CNTR":u32, "QE.STAT"=→"ENC.C_0.STAT":u8)  [unwired: 11 in]
    n200 = call "DIO 1-bit.vi"("DIR"=w489, "OUT"=w495, "DIO Refnum"=refnum<k21> "ConnectorC/DIO1") -> ("IN"=w482:bool)  [unwired: 8 in]
    n201 = call "DIO_PWM.vi"("DIO.OUT"=w494, "DIO.DIR"=w488, "PWM.CS"="PWM.C_0.CS", "PWM.CNFG"="PWM.C_0.CNFG", "PWM.CMP"="PWM.C_0.CMP", "PWM.MAX"="PWM.C_0.MAX", "DIO/PWM"=refnum<k21> "ConnectorC/DIO3", "SELECT"=w500) -> ("DIO.IN"=w481:bool, "PWM.CNTR"=→"PWM.C_0.CNTR":u16)  [unwired: 10 in]
    n202 = call "DIO_Encoder.vi"("DIO.1:0.OUT"=w493, "DIO.1:0.DIR"=w487, "QE.CNFG"=u8 1, "DIO.1/QE.B"=refnum<k21> "ConnectorC/DIO6", "SELECT"=TRUE, "DIO.0/QE.A"=refnum<k21> "ConnectorC/DIO4") -> ("DIO.1:0.IN"=w480:fxp<+,2,2>, "QE.CNTR"=→"ENC.C_1.CNTR":u32, "QE.STAT"=→"ENC.C_1.STAT":u8)  [unwired: 11 in]
    n203 = call "DIO 1-bit.vi"("DIR"=w486, "OUT"=w492, "DIO Refnum"=refnum<k21> "ConnectorC/DIO5") -> ("IN"=w479:bool)  [unwired: 8 in]
    n204 = call "DIO_PWM.vi"("DIO.OUT"=w491, "DIO.DIR"=w485, "PWM.CS"="PWM.C_1.CS", "PWM.CNFG"="PWM.C_1.CNFG", "PWM.CMP"="PWM.C_1.CMP", "PWM.MAX"="PWM.C_1.MAX", "DIO/PWM"=refnum<k21> "ConnectorC/DIO7", "SELECT"=w499) -> ("DIO.IN"=w478:bool, "PWM.CNTR"=→"PWM.C_1.CNTR":u16)  [unwired: 10 in]
    n205 = call "Join myDAQ DIO.vi"("IN 7"=w478, "IN 5"=w479, "IN 6, IN 4"=w480, "IN 2, IN 0"=w483, "IN 3"=w481, "IN 1"=w482) -> ("IN 7:0"=→"DIO.C_7:0.IN":u8)  [unwired: 4 in]
  }
  n206 = node-c288(w10) -> ()
